vi "DSK1.vi"(11 "file path (dialog if empty)":path) -> (0 "Money":dbl[](array[numeric]), 1 "Transfers 1":string[](array[string]), 2 "Transfers 2":string[](array[string]), 3 "Transfers":string[][](array[string]), 4 "Enum":T1(ring))   [LabVIEW 2023]
uses:
  <vilib>/Utility/file.llb/Read Delimited Spreadsheet (string).vi
panel:
  out "Array":string[](array[string])
  out "Concatenated string":string
  out "all rows":string[][](array[string])
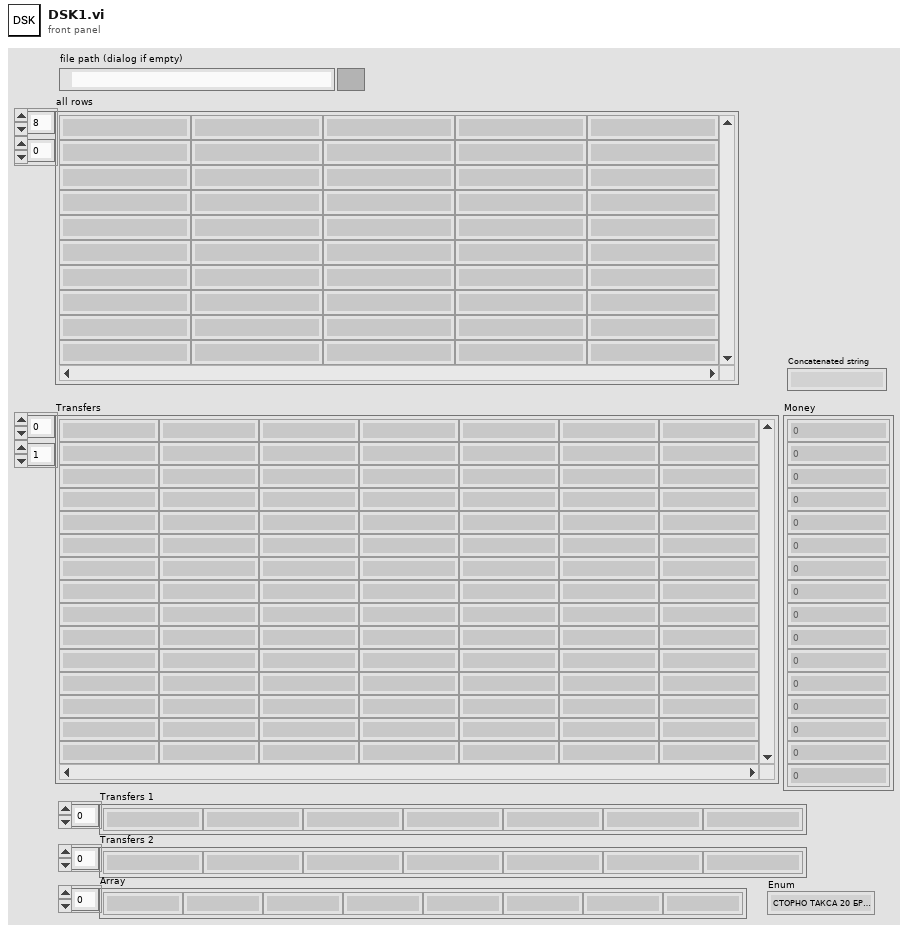
[diagram p1: front panel]
types:
  T1 = enum16{"СТОРНО ТАКСА 20 БР.SMS/VIBER", "ТРАНСФЕР МЕЖДУ СВОИ СМЕТКИ", "ПЛАТЕНА ЛИХВА ОВЪРДРАФТ", "АВАНС08.2024 СПИСЪК 070662255700 КЛОН 0605", "ТАКСА ПАКЕТНО ОБСЛУЖВАНЕ", "ТАКСА ЗА 51 БР.SMS/VIBER", "516849xxxxxx5165 ТЕГЛЕНЕ НА ATM 26.07.2024 19:38", "516849xxxxxx5165 ТЕГЛЕНЕ НА ATM 17.07.2024 22:20", "D0004737071200731 7501123464 КЪМ CK-0000000010592240", "ПЛАЩАНЕ ПО ЗАЕМ КЪМ PL-0000000027262271", "516849xxxxxx5165 ТЕГЛЕНЕ НА ATM 13.07.2024 09:57", "516849xxxxxx5165 ТЕГЛЕНЕ НА ATM 13.07.2024 10:48", "BREZOVO", "TРАНСФЕР МЕЖДУ СВОИ СМЕТКИ", "15.07.2024 ЕЛ ЕНЕРГИЯ АБ.N. 1000321755", "15.07.2024 ЕЛ ЕНЕРГИЯ АБ.N. 310254419035 Ф-РА N: 380203882/10.07.24", "15.07.2024 ТЕЛЕКОМУНИКАЦИЯ АБ.N. 14724468001 БЛАГОЙ НИКОЛОВ НИКОЛО", "БЛАГОДАРЯ", "ЗАПЛАТА06.2024 СПИСЪК 070662255701 КЛОН 0605", "NCC WITHDRAWAL", "516849xxxxxx5165 ТЕГЛЕНЕ НА ATM 04.07.2024 10:49", "516849xxxxxx5165 ТЕГЛЕНЕ НА ATM 29.06.2024 09:54", "516849xxxxxx5165 ТЕГЛЕНЕ НА ATM 29.06.2024 09:52", "АВАНС07.2024 СПИСЪК 070662255700 КЛОН 0605", "НЯМА", "ТАКСА ЗА 24 БР.SMS/VIBER НАТРУПАН ОБЩ БР. SMS 44", "28.06.2024 ИНТЕРНЕТ АБ.N. 10221645 НЕТ-СЪРФ.НЕТ ЕООД", "28.06.2024 ЕЛ ЕНЕРГИЯ АБ.N. 1225769 ЕВН БЪЛГАРИЯ ЕЛЕКТРОСНАБДЯВАНЕ", "28.06.2024 ЕЛ ЕНЕРГИЯ АБ.N. 1000321755 ЕВН БЪЛГАРИЯ ЕЛЕКТРОСНАБДЯВАНЕ", "516849xxxxxx5165 ТЕГЛЕНЕ НА ATM 25.06.2024 06:59", "516849xxxxxx5165 ПЛАЩАНЕ НА ПОС 22.06.2024 14:34", "СБКО106.2024 СПИСЪК 200662255704 КЛОН 0605", "18.06.2024 ТЕЛЕКОМУНИКАЦИЯ АБ.N. 14724468001 VIVACOM", "18.06.2024 ЕЛ ЕНЕРГИЯ АБ.N. 310254419035 ЕЛЕКТРОХОЛД ПРОДАЖБИ АД", "516849xxxxxx5165 ТЕГЛЕНЕ НА ATM 17.06.2024 07:00", "ЗАПЛАТА05.2024 СПИСЪК 070662255701 КЛОН 0605", "516849xxxxxx5165 ТЕГЛЕНЕ НА ATM 11.06.2024 19:22", "516849xxxxxx5165 ТЕГЛЕНЕ НА ATM 10.06.2024 07:06", "516849xxxxxx5165 ТЕГЛЕНЕ НА ATM 10.06.2024 07:07", "516849xxxxxx5165 ТЕГЛЕНЕ НА ATM 05.06.2024 07:05", "05.06.2024 ЕЛ ЕНЕРГИЯ АБ.N. 1225769 ЕВН БЪЛГАРИЯ ЕЛЕКТРОСНАБДЯВАНЕ", "05.06.2024 ИНТЕРНЕТ АБ.N. 10221645 НЕТ-СЪРФ.НЕТ ЕООД", "АВАНС06.2024 СПИСЪК 070662255700 КЛОН 0605", "ЧАСОВНИК", "ТАКСА ЗА 17 БР.SMS/VIBER НАТРУПАН ОБЩ БР. SMS 37", "516849xxxxxx5165 ТЕГЛЕНЕ НА ATM 26.05.2024 17:04", "516849xxxxxx5165 ТЕГЛЕНЕ НА ATM 17.05.2024 13:48", "516849xxxxxx5165 ТЕГЛЕНЕ НА ATM 16.05.2024 10:23", "516849xxxxxx5165 ТЕГЛЕНЕ НА ATM 16.05.2024 06:54", "15.05.2024 ЕЛ ЕНЕРГИЯ АБ.N. 1000321755 ЕВН БЪЛГАРИЯ ЕЛЕКТРОСНАБДЯВАНЕ", "15.05.2024 ЕЛ ЕНЕРГИЯ АБ.N. 310254419035 ЕЛЕКТРОХОЛД ПРОДАЖБИ АД", "ЗАПЛАТА04.2024 СПИСЪК 070662255705 КЛОН 0605", "516849xxxxxx5165 ТЕГЛЕНЕ НА ATM 13.05.2024 19:50", "09.05.2024 ИНТЕРНЕТ АБ.N. 10221645 НЕТ-СЪРФ.НЕТ ЕООД", "09.05.2024 ТЕЛЕКОМУНИКАЦИЯ АБ.N. 14724468001 VIVACOM", "09.05.2024 ЕЛ ЕНЕРГИЯ АБ.N. 1225769 ЕВН БЪЛГАРИЯ ЕЛЕКТРОСНАБДЯВАНЕ", "516849xxxxxx5165 ТЕГЛЕНЕ НА ATM 06.05.2024 12:22", "СБКО104.2024 СПИСЪК 200662255701 КЛОН 0605", "АВАНС05.2024 СПИСЪК 070662255700 КЛОН 0605", "516849xxxxxx5165 ПЛАЩАНЕ НА ПОС 29.04.2024 13:53", "516849xxxxxx5165 ПЛАЩАНЕ НА ПОС 29.04.2024 13:38", "516849xxxxxx5165 ПЛАЩАНЕ НА ПОС 29.04.2024 13:48", "ТАКСА ЗА 19 БР.SMS/VIBER НАТРУПАН ОБЩ БР. SMS 39", "516849xxxxxx5165 ТЕГЛЕНЕ НА ATM 24.04.2024 07:03", "516849xxxxxx5165 ТЕГЛЕНЕ НА ATM 20.04.2024 10:51", "516849xxxxxx5165 ТЕГЛЕНЕ НА ATM 16.04.2024 15:25", "15.04.2024 ЕЛ ЕНЕРГИЯ АБ.N. 310254419035 Ф-РА N: 375024781/10.04.24", "15.04.2024 ТЕЛЕКОМУНИКАЦИЯ АБ.N. 14724468001 БЛАГОЙ НИКОЛОВ НИКОЛО", "15.04.2024 ЕЛ ЕНЕРГИЯ АБ.N. 1000321755", "ЗАПЛАТА03.2024 СПИСЪК 070662255701 КЛОН 0605", "516849xxxxxx5165 ТЕГЛЕНЕ НА ATM 06.04.2024 09:48", "516849xxxxxx5165 ТЕГЛЕНЕ НА ATM 03.04.2024 15:20", "04.04.2024 ЕЛ ЕНЕРГИЯ АБ.N. 1225769 ЕВН БЪЛГАРИЯ ЕЛЕКТРОСНАБДЯВАНЕ", "04.04.2024 ИНТЕРНЕТ АБ.N. 10221645 НЕТ-СЪРФ.НЕТ ЕООД", "516849xxxxxx5165 ТЕГЛЕНЕ НА ATM 02.04.2024 15:14", "516849xxxxxx5165 ТЕГЛЕНЕ НА ATM 02.04.2024 15:13", "АВАНС04.2024 СПИСЪК 070662255700 КЛОН 0605", "516849xxxxxx5165 ТЕГЛЕНЕ НА ATM 28.03.2024 15:27", "516849xxxxxx5165 ТЕГЛЕНЕ НА ATM 28.03.2024 15:30", "ТАКСА ЗА 26 БР.SMS/VIBER НАТРУПАН ОБЩ БР. SMS 46", "516849xxxxxx5165 ТЕГЛЕНЕ НА ATM 20.03.2024 13:44", "516849xxxxxx5165 ТЕГЛЕНЕ НА ATM 19.03.2024 15:13", "18.03.2024 ЕЛ ЕНЕРГИЯ АБ.N. 1225769 ЕВН БЪЛГАРИЯ ЕЛЕКТРОСНАБДЯВАНЕ", "18.03.2024 ЕЛ ЕНЕРГИЯ АБ.N. 1000321755 ЕВН БЪЛГАРИЯ ЕЛЕКТРОСНАБДЯВАНЕ", "16.03.2024 ЕЛ ЕНЕРГИЯ АБ.N. 310254419035 ЕЛЕКТРОХОЛД ПРОДАЖБИ АД", "ЗАПЛАТА02.2024 СПИСЪК 070662255706 КЛОН 0605", "12.03.2024 ТЕЛЕКОМУНИКАЦИЯ АБ.N. 14724468001 VIVACOM", "11.03.2024 ИНТЕРНЕТ АБ.N. 10221645 НЕТ-СЪРФ.НЕТ ЕООД", "516849xxxxxx5165 ТЕГЛЕНЕ НА ATM 06.03.2024 15:03", "516849xxxxxx5165 ТЕГЛЕНЕ НА ATM 03.03.2024 16:57", "516849xxxxxx5165 ТЕГЛЕНЕ НА ATM 03.03.2024 16:56", "516849xxxxxx5165 ТЕГЛЕНЕ НА ATM 03.03.2024 16:55", "СБКО102.2024 СПИСЪК 200662255701 КЛОН 0605", "АВАНС03.2024 СПИСЪК 070662255700 КЛОН 0605", "ТАКСА ЗА 20 БР.SMS/VIBER НАТРУПАН ОБЩ БР. SMS 40", "516849xxxxxx5165 ТЕГЛЕНЕ НА ATM 21.02.2024 16:30", "516849xxxxxx5165 ТЕГЛЕНЕ НА ATM 17.02.2024 10:19", "19.02.2024 ЕЛ ЕНЕРГИЯ АБ.N. 310254419035 ЕЛЕКТРОХОЛД ПРОДАЖБИ АД", "19.02.2024 ТЕЛЕКОМУНИКАЦИЯ АБ.N. 14724468001 VIVACOM", "19.02.2024 ЕЛ ЕНЕРГИЯ АБ.N. 1225769 ЕВН БЪЛГАРИЯ ЕЛЕКТРОСНАБДЯВАНЕ", "19.02.2024 ЕЛ ЕНЕРГИЯ АБ.N. 1000321755 ЕВН БЪЛГАРИЯ ЕЛЕКТРОСНАБДЯВАНЕ", "ЗАПЛАТА01.2024 СПИСЪК 070662255703 КЛОН 0605", "516849xxxxxx5165 ТЕГЛЕНЕ НА ATM 14.02.2024 08:38", "516849xxxxxx5165 ТЕГЛЕНЕ НА ATM 12.02.2024 14:49", "12.02.2024 ИНТЕРНЕТ АБ.N. 10221645 НЕТ-СЪРФ.НЕТ ЕООД", "АВАНС02.2024 СПИСЪК 070662255700 КЛОН 0605", "ТАКСА ЗА 32 БР.SMS/VIBER ЗА 01.24 И НЕСЪБРАНИ ЗА 12.23 НАТРУПАН ОБЩ БР. SMS 52", "516849xxxxxx5165 ТЕГЛЕНЕ НА ATM 27.01.2024 13:24", "516849xxxxxx5165 ТЕГЛЕНЕ НА ATM 24.01.2024 15:36", "516849xxxxxx5165 ТЕГЛЕНЕ НА ATM 23.01.2024 10:02", "516849xxxxxx5165 ТЕГЛЕНЕ НА ATM 19.01.2024 18:56", "516849xxxxxx5165 ТЕГЛЕНЕ НА ATM 17.01.2024 16:18", "516849xxxxxx5165 ТЕГЛЕНЕ НА ATM 14.01.2024 15:52", "15.01.2024 ЕЛ ЕНЕРГИЯ АБ.N. 310254419035 ЕЛЕКТРОХОЛД ПРОДАЖБИ АД", "ЗАПЛАТА12.2023 СПИСЪК 070662255703 КЛОН 0605", "516849xxxxxx5165 ТЕГЛЕНЕ НА ATM 11.01.2024 12:04", "11.01.2024 ТЕЛЕКОМУНИКАЦИЯ АБ.N. 14724468001 VIVACOM", "11.01.2024 ЕЛ ЕНЕРГИЯ АБ.N. 1225769 ЕВН БЪЛГАРИЯ ЕЛЕКТРОСНАБДЯВАНЕ", "11.01.2024 ЕЛ ЕНЕРГИЯ АБ.N. 1000321755 ЕВН БЪЛГАРИЯ ЕЛЕКТРОСНАБДЯВАНЕ", "11.01.2024 ИНТЕРНЕТ АБ.N. 10221645 НЕТ-СЪРФ.НЕТ ЕООД", "516849xxxxxx5165 ПЛАЩАНЕ НА ПОС 29.12.2023 14:49", "516849xxxxxx5165 ТЕГЛЕНЕ НА ATM 01.01.2024 12:52", "516849xxxxxx5165 ТЕГЛЕНЕ НА ATM 01.01.2024 12:51", "АВАНС01.2024 СПИСЪК 070662255700 КЛОН 0605", "516849xxxxxx5165 ПЛАЩАНЕ НА ПОС 28.12.2023 13:59", "516849xxxxxx5165 ПЛАЩАНЕ НА ПОС 28.12.2023 15:38", "516849xxxxxx5165 ПЛАЩАНЕ НА ПОС 24.12.2023 12:03", "516849xxxxxx5165 ПЛАЩАНЕ НА ПОС 24.12.2023 12:23", "516849xxxxxx5165 ПЛАЩАНЕ НА ПОС 28.12.2023 12:34", "516849xxxxxx5165 ПЛАЩАНЕ НА ПОС 24.12.2023 12:13", "516849xxxxxx5165 ПЛАЩАНЕ НА ПОС 24.12.2023 12:09", "516849xxxxxx5165 ПЛАЩАНЕ НА ПОС 24.12.2023 12:39", "516849xxxxxx5165 ТЕГЛЕНЕ НА ATM 21.12.2023 17:22", "516849xxxxxx5165 ТЕГЛЕНЕ НА ATM 21.12.2023 07:05", "516849xxxxxx5165 ТЕГЛЕНЕ НА ATM 20.12.2023 17:12", "516849xxxxxx5165 ТЕГЛЕНЕ НА ATM 19.12.2023 07:00", "516849xxxxxx5165 ПЛАЩАНЕ НА ПОС 18.12.2023 12:27", "516849xxxxxx5165 ТЕГЛЕНЕ НА ATM 15.12.2023 17:28", "15.12.2023 ЕЛ ЕНЕРГИЯ АБ.N. 1000321755", "15.12.2023 ЕЛ ЕНЕРГИЯ АБ.N. 310254419035 ЕЛЕКТРОХОЛД ПРОДАЖБИ АД", "15.12.2023 ТЕЛЕКОМУНИКАЦИЯ АБ.N. 14724468001 VIVACOM", "15.12.2023 ЕЛ ЕНЕРГИЯ АБ.N. 1225769 ЕВН БЪЛГАРИЯ ЕЛЕКТРОСНАБДЯВАНЕ", "15.12.2023 ИНТЕРНЕТ АБ.N. 10221645 НЕТ-СЪРФ.НЕТ ЕООД", "516849xxxxxx5165 ТЕГЛЕНЕ НА ATM 14.12.2023 07:11", "ЗАПЛАТА11.2023 СПИСЪК 070662255701 КЛОН 0605", "516849xxxxxx5165 ТЕГЛЕНЕ НА ATM 11.12.2023 07:13", "516849xxxxxx5165 ТЕГЛЕНЕ НА ATM 08.12.2023 17:42", "516849xxxxxx5165 ТЕГЛЕНЕ НА ATM 07.12.2023 07:10", "516849xxxxxx5165 ТЕГЛЕНЕ НА ATM 05.12.2023 07:06", "АВАНС12.2023 СПИСЪК 070662255700 КЛОН 0605", "ТАКСА ЗА 11.10-30.11.2023г. 48 БР.SMS/VIBER НАТРУПАН ОБЩ БР. SMS 68", "516849xxxxxx5165 ТЕГЛЕНЕ НА ATM 26.11.2023 15:03", "516849xxxxxx5165 ТЕГЛЕНЕ НА ATM 23.11.2023 07:12", "516849xxxxxx5165 ПЛАЩАНЕ НА ПОС 20.11.2023 15:15", "516849xxxxxx5165 ТЕГЛЕНЕ НА ATM 20.11.2023 08:44", "516849xxxxxx5165 ТЕГЛЕНЕ НА ATM 15.11.2023 07:08", "15.11.2023 ЕЛ ЕНЕРГИЯ АБ.N. 310254419035 ЕЛЕКТРОХОЛД ПРОДАЖБИ АД", "15.11.2023 ТЕЛЕКОМУНИКАЦИЯ АБ.N. 14724468001 VIVACOM", "ЗАПЛАТА10.2023 СПИСЪК 070662255701 КЛОН 0605", "516849xxxxxx5165 ТЕГЛЕНЕ НА ATM 13.11.2023 07:04", "516849xxxxxx5165 ТЕГЛЕНЕ НА ATM 10.11.2023 17:28", "516849xxxxxx5165 ТЕГЛЕНЕ НА ATM 13.11.2023 07:05", "516849xxxxxx5165 ТЕГЛЕНЕ НА ATM 08.11.2023 06:53", "516849xxxxxx5165 ТЕГЛЕНЕ НА ATM 06.11.2023 09:06", "516849xxxxxx5165 ПЛАЩАНЕ НА ПОС 03.11.2023 11:17", "516849xxxxxx5165 ТЕГЛЕНЕ НА ATM 03.11.2023 14:50", "01.11.2023 ЕЛ ЕНЕРГИЯ АБ.N. 310254419035 ЕЛЕКТРОХОЛД ПРОДАЖБИ АД", "01.11.2023 ИНТЕРНЕТ АБ.N. 10221645 НЕТ-СЪРФ.НЕТ ЕООД", "01.11.2023 ЕЛ ЕНЕРГИЯ АБ.N. 1225769 ЕВН БЪЛГАРИЯ ЕЛЕКТРОСНАБДЯВАНЕ", "01.11.2023 ТЕЛЕКОМУНИКАЦИЯ АБ.N. 14724468001 VIVACOM", "АВАНС11.2023 СПИСЪК 070662255700 КЛОН 0605", "516849xxxxxx5165 ТЕГЛЕНЕ НА ATM 28.10.2023 14:04", "516849xxxxxx5165 ТЕГЛЕНЕ НА ATM 27.10.2023 06:45", "516849xxxxxx5165 ТЕГЛЕНЕ НА ATM 25.10.2023 06:49", "516849xxxxxx5165 ТЕГЛЕНЕ НА ATM 21.10.2023 09:14", "516849xxxxxx5165 ТЕГЛЕНЕ НА ATM 19.10.2023 06:57", "HONDA", "516849xxxxxx5165 ПЛАЩАНЕ НА ПОС 16.10.2023 11:47", "516849xxxxxx5165 ТЕГЛЕНЕ НА ATM 16.10.2023 06:55", "516849xxxxxx5165 ТЕГЛЕНЕ НА ATM 12.10.2023 16:35", "ЗАПЛАТА09.2023 СПИСЪК 070662255703 КЛОН 0605", "516849xxxxxx5165 ТЕГЛЕНЕ НА ATM 10.10.2023 07:05", "08.10.2023 ИНТЕРНЕТ АБ.N. 10221645 НЕТ-СЪРФ.НЕТ ЕООД", "08.10.2023 ЕЛ ЕНЕРГИЯ АБ.N. 1225769 ЕВН БЪЛГАРИЯ ЕЛЕКТРОСНАБДЯВАНЕ", "516849xxxxxx5165 ТЕГЛЕНЕ НА ATM 05.10.2023 06:53", "516849xxxxxx5165 ТЕГЛЕНЕ НА ATM 04.10.2023 07:07", "АВАНС10.2023 СПИСЪК 070662255700 КЛОН 0605", "516849xxxxxx5165 ТЕГЛЕНЕ НА ATM 29.09.2023 07:04", "516849xxxxxx5165 ТЕГЛЕНЕ НА ATM 26.09.2023 16:35", "516849xxxxxx5165 ТЕГЛЕНЕ НА ATM 25.09.2023 18:07", "516849xxxxxx5165 ТЕГЛЕНЕ НА ATM 25.09.2023 11:45", "ПОЛИЦА: 440223213004410 АВТОКАСКО - PB9134TA", "516849xxxxxx5165 ТЕГЛЕНЕ НА ATM 19.09.2023 17:16", "516849xxxxxx5165 ТЕГЛЕНЕ НА ATM 14.09.2023 16:28", "516849xxxxxx5165 ТЕГЛЕНЕ НА ATM 14.09.2023 07:12", "14.09.2023 ЕЛ ЕНЕРГИЯ АБ.N. 310254419035 ЕЛЕКТРОХОЛД ПРОДАЖБИ АД", "14.09.2023 ТЕЛЕКОМУНИКАЦИЯ АБ.N. 14724468001 VIVACOM", "ЗАПЛАТА08.2023 СПИСЪК 070662255703 КЛОН 0605", "516849xxxxxx5165 ТЕГЛЕНЕ НА ATM 12.09.2023 16:57", "10.09.2023 ИНТЕРНЕТ АБ.N. 10221645 НЕТ-СЪРФ.НЕТ ЕООД", "10.09.2023 ЕЛ ЕНЕРГИЯ АБ.N. 1225769 ЕВН БЪЛГАРИЯ ЕЛЕКТРОСНАБДЯВАНЕ", "516849xxxxxx5165 ТЕГЛЕНЕ НА ATM 07.09.2023 16:57", "516849xxxxxx5165 ТЕГЛЕНЕ НА ATM 02.09.2023 21:57", "СБКО108.2023 СПИСЪК 200662255701 КЛОН 0605", "516849xxxxxx5165 ТЕГЛЕНЕ НА ATM 31.08.2023 17:03", "АВАНС09.2023 СПИСЪК 070662255700 КЛОН 0605", "ТАКСА ЗА 35 БР.SMS/VIBER НАТРУПАН ОБЩ БР. SMS 55", "516849xxxxxx5165 ТЕГЛЕНЕ НА ATM 29.08.2023 16:59", "516849xxxxxx5165 ТЕГЛЕНЕ НА ATM 25.08.2023 13:45", "ОБМЕН НА ВАЛУТА", "516849xxxxxx5165 ТЕГЛЕНЕ НА ATM 22.08.2023 10:43", "516849xxxxxx5165 ТЕГЛЕНЕ НА ATM 21.08.2023 16:56", "БРОЕНА СУМА КЛИЕНТ ПРЕМИУЧ 7501123464/652391565", "Ш.30011", "14.08.2023 ИНТЕРНЕТ АБ.N. 10221645", "14.08.2023 ТЕЛЕКОМУНИКАЦИЯ АБ.N. 14724468001 БЛАГОЙ НИКОЛОВ НИКОЛО", "14.08.2023 ЕЛ ЕНЕРГИЯ АБ.N. 310254419035 Ф-РА N: 361375930/09.08.23", "14.08.2023 ЕЛ ЕНЕРГИЯ АБ.N. 1225769", "ЗАПЛАТА07.2023 СПИСЪК 070662255702 КЛОН 0605", "516849xxxxxx5165 ТЕГЛЕНЕ НА ATM 09.08.2023 09:56", "188311"}
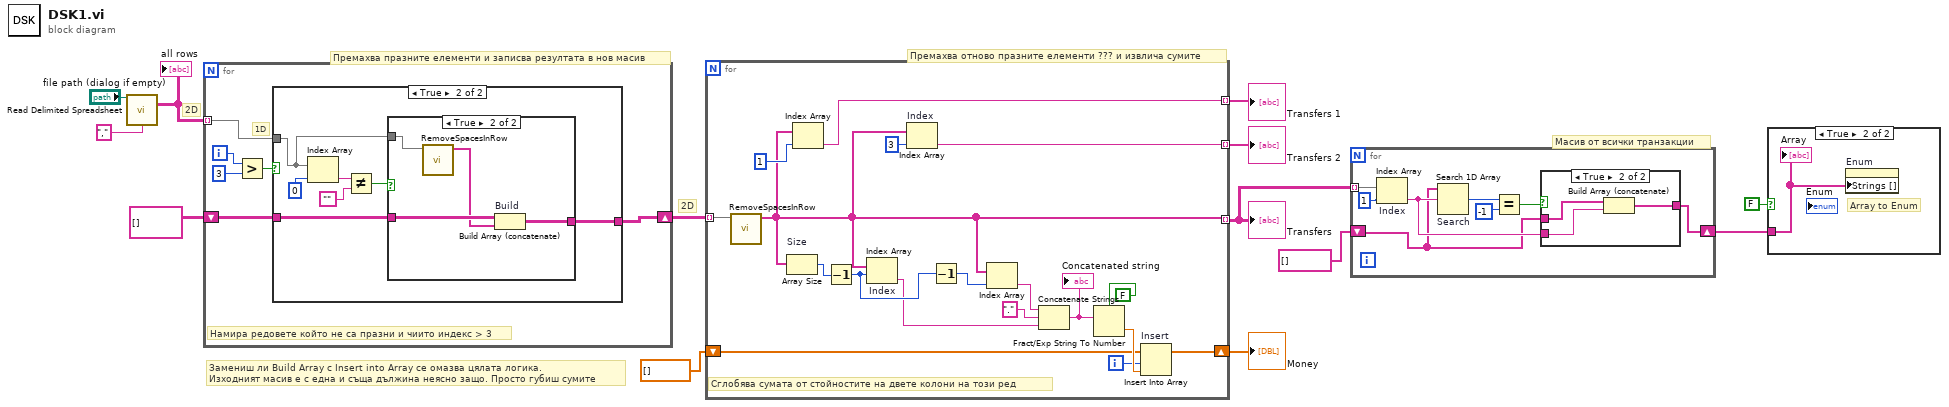
[diagram p0: block diagram]
diagram:
  # "Масив от всички транзакции"
  # "2D"
  # "2D"
  # "Замениш ли Build Array с Insert into Array се омазва цялата логика.\nИзходният масив е с една и съща дължина неясно защо. Просто губиш сумите"
  # "Премахва отново празните елементи ??? и извлича сумите"
  # "Премахва празните елементи и записва резултата в нов масив"
  n1 = call-poly <vilib>:"Read Delimited Spreadsheet.vi"("file path (dialog if empty)"="file path (dialog if empty)", "delimiter (\\t)"="," ("delimiter (\\t)")) -> ("all rows"=w12:string[][])  [unwired: 8 in, 5 out]
  "all rows" <- w12
  n2 = for {
    tunnel: w12 -> [w16] mode=indexing
    shift-right: [w14] -> w9
    shift-left: string[][] [] -> [w15]
    i -> [w19]
    # "Намира редовете който не са празни и чиито индекс > 3"
    # "1D"
    n3 = Greater?(x=w19, y=3) -> (0:w17:bool)
    n4 = case shown="True" w17 {
      tunnel: w16 -> [_ w23]
      tunnel: w15 -> [w20 w22]
      tunnel: [w20 w21] -> w14
      frame False {
      }
      frame True {
        n5 = Index Array "Index Array"(array=w23, index=0 ("y")) -> (element=w26:string)
        n6 = Not Equal?(x=w26, y="") -> (x != y?=w24:bool)
        n7 = case shown="True" w24 {
          tunnel: w23 -> [_ w32]
          tunnel: w22 -> [w28 w31]
          tunnel: [w28 w30] -> w21
          frame False {
          }
          frame True {
            n8 = call "RemoveSpacesInRow.vi"("Array"=w32) -> ("outArray"=w29:string[])  [unwired: 10 in]
            n9 = Build Array (concatenate) "Build"(w31, w29) -> (w30:string[][])
          }
        }
      }
    }
  }
  n10 = for {
    tunnel: w9 -> [w50] mode=indexing
    tunnel: [w37] -> w4 mode=indexing
    shift-right: [w41] -> w7
    shift-left: dbl[] [] -> [w40]
    tunnel: [w36] -> w5 mode=indexing
    tunnel: [w35] -> w6 mode=indexing
    i -> [w42]
    # "Сглобява сумата от стойностите на двете колони на този ред"
    n11 = call "RemoveSpacesInRow.vi"("Array"=w50) -> ("outArray"=w37:string[])  [unwired: 10 in]
    n12 = Array Size "Size"(array=w37) -> (size(s)=w47:i32)
    n13 = Index Array(array=w37, index=1) -> (element=w36:string)
    n14 = Decrement(x=w47) -> (x-1=w46:i32)
    n15 = Index Array "Index"(array=w37, index=w46) -> (element=w45:string)
    n16 = Index Array "Index"(array=w37, index=3) -> (element=w35:string)
    n17 = Decrement(x=w46) -> (x-1=w49:i32)
    n18 = Index Array(array=w37, index=w49) -> (element=w48:string)
    n19 = Concatenate Strings(w48, ".", w45) -> (w34:string)
    "Concatenated string" <- w34
    n20 = Fract/Exp String To Number(use system decimal point (T)=FALSE, string=w34) -> (number=w43:dbl)  [unwired: 2 in, 1 out]
    n21 = Insert Into Array "Insert"(array=w40, index=w42, new element=w43) -> (w41:dbl[])
  }
  "Transfers" <- w4
  "Money" <- w7
  "Transfers 2" <- w6
  "Transfers 1" <- w5
  n22 = for {
    tunnel: w4 -> [w58] mode=indexing
    shift-right: [w52] -> w2
    shift-left: string[] [] -> [w51]
    n23 = Index Array "Index"(array=w58, index=1) -> (element=w53:string)
    n24 = Search 1D Array "Search"(1D array=w51, element=w53) -> (index of element=w56:i32)  [unwired: 1 in]
    n25 = Equal?(x=w56, y=-1) -> (x = y?=w54:bool)
    n26 = case shown="True" w54 {
      tunnel: w53 -> [_ w62]
      tunnel: [w59 w61] -> w52
      tunnel: w51 -> [w59 w60]
      frame False {
      }
      frame True {
        n27 = Build Array (concatenate)(w60, w62) -> (w61:string[])
      }
    }
  }
  n28 = case shown="True" FALSE {
    tunnel: w2 -> [_ w63]
    frame False {
    }
    frame True {
      # "Array to Enum"
      n29 = property on="Enum" class="Enum (strict)"("Strings []"=w63) -> ()  [unwired: 2 in, 2 out]
      "Array" <- w63
    }
  }
